vi "HRR-Reorder.vi"(10 "In":dbl[][](array[numeric])) -> (2 "Out":dbl[][](array[numeric]))   [LabVIEW 2019]
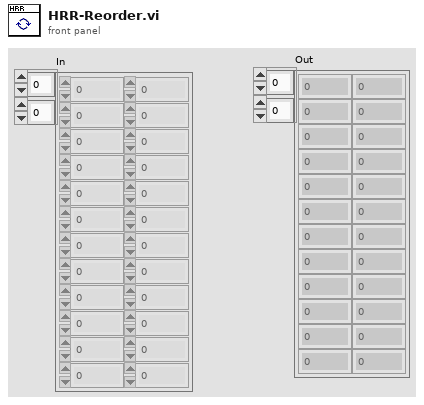
[diagram p1: front panel]
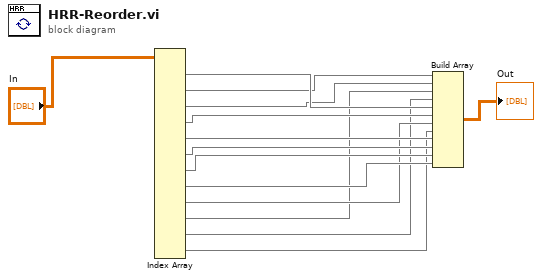
[diagram p0: block diagram]
diagram:
  n1 = Index Array(array="In") -> (element #1=w12:dbl[], element #2=w11:dbl[], element #3=w10:dbl[], element #4=w9:dbl[], element #5=w8:dbl[], element #6=w7:dbl[], element #7=w6:dbl[], element #8=w5:dbl[], element #9=w4:dbl[], element #10=w3:dbl[], element #11=w2:dbl[], element #12=w1:dbl[])  [unwired: 24 in]
  n2 = Build Array(w11, w10, w3, w2, w12, w9, w4, w1, w8, w7, w6, w5) -> (→"Out":dbl[][])
